vi "Send Measurement Done.vi"(8 "error in (no error)":errorcluster, 10 "Unique Identifier":string, 11 "Message Enqueuer in":refnum<class "Message Enqueuer.lvclass">) -> (3 "Message Enqueuer out":refnum<class "Message Enqueuer.lvclass">)   [LabVIEW 2026, in "Controller Actor.lvlib" / "Measurement Done.lvclass"]
uses:
  Measurement Done.lvclass
  Measurement Done.lvclass/Measurement Done.ctl
  <vilib>/ActorFramework/Message Enqueuer/Message Enqueuer.lvclass
panel:
  out "error out":errorcluster
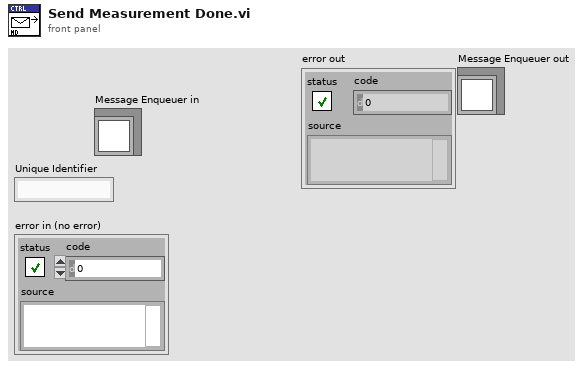
[diagram p1: front panel]
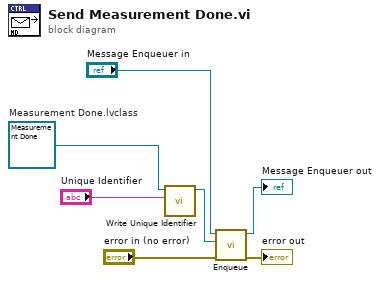
[diagram p0: block diagram]
diagram:
  w7 = refnum<class "Measurement Done.lvclass"> refnum  # Measurement Done.lvclass
  n1 = call "Write Unique Identifier.vi"("Unique Identifier"="Unique Identifier", "Measurement Done in"=w7) -> ("Measurement Done out"=w5:refnum<class "Measurement Done.lvclass">)  [unwired: 8 in, 1 out]
  n2 = call <vilib>:"Enqueue.vi"("error in (no error)"="error in (no error)", "Message"=w5, "Message Enqueuer in"="Message Enqueuer in") -> ("error out"=→"error out":errorcluster, "Message Enqueuer out"=→"Message Enqueuer out":refnum<class "Message Enqueuer.lvclass">)  [unwired: 7 in]
